vi "playground.vi"() -> ()   [LabVIEW 2014]
panel:
  out "Q Meter":cluster{"Y":dbl[], "Y":dbl[]}[](graph)
  out "Modulator":dynamicdata(graph)
  out "Triangle Waveform":dynamicdata(graph)
  in  "# sweeps":dbl
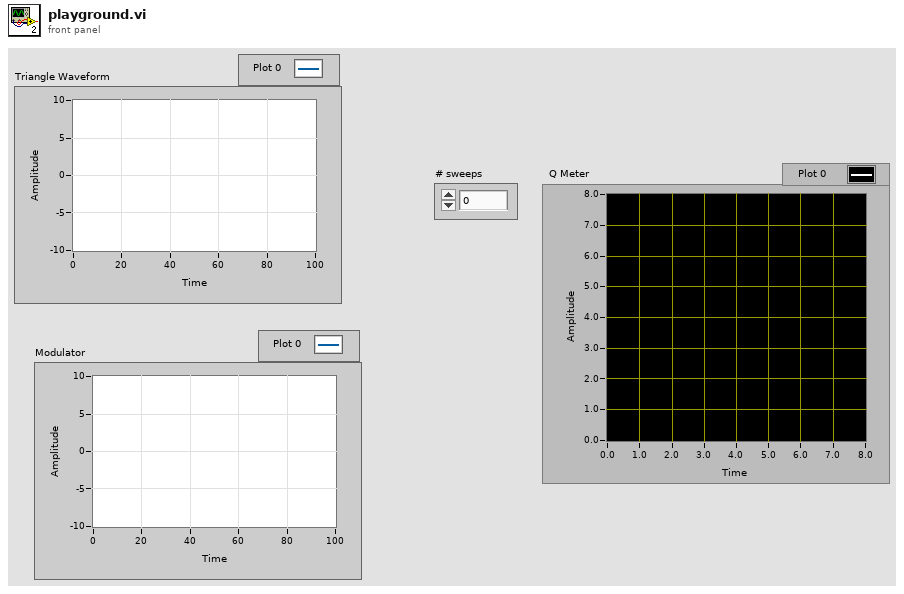
[diagram p1: front panel]
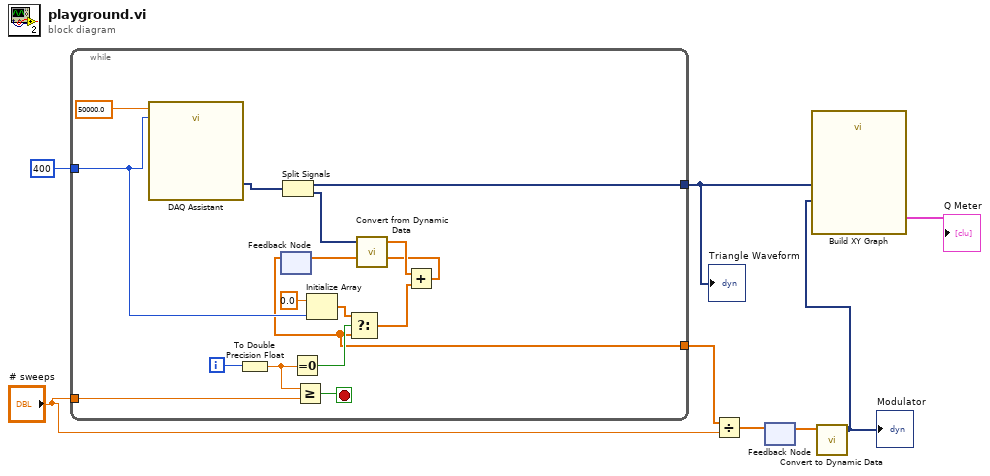
[diagram p0: block diagram]
diagram:
  n1 = while {
    tunnel: 400 -> [w16]
    tunnel: "# sweeps" -> [w12]
    tunnel: [w10] -> w6
    tunnel: [w9] -> w5
    i -> [w15]
    stop <- w13 stop-if-true
    n2 = call "DAQ Assistant"("rate"=50000.0, "number of samples"=w16) -> ("data"=w23:dynamicdata)  [unwired: 15 in, 2 out]
    n3 = To Double Precision Float(number=w15) -> (double precision float=w11:dbl)
    n4 = feedback #1() -> (w9:dbl[])  [unwired: 1 in]
    n5 = Split Signals(w23) -> (w10:dynamicdata, w22:dynamicdata)  [unwired: 2 in]
    n6 = Equal To 0?(x=w11) -> (x = 0?=w14:bool)
    n7 = Greater Or Equal?(x=w11, y=w12) -> (x >= y?=w13:bool)
    n8 = Initialize Array(0.0, w16) -> (w19:dbl[])
    n9 = Select(t=w19, s=w14, f=w9) -> (s? t:f=w17:dbl[])
    n10 = call "Convert from Dynamic Data"("Dynamic Data Type"=w22) -> ("Array"=w21:dbl[])  [unwired: 3 in]
    n11 = Add(x=w21, y=w17) -> (x+y=w20:dbl[])
    n12 = feedback-in #1(w20) -> ()
  }
  "Triangle Waveform" <- w6
  n13 = Divide(x=w5, y="# sweeps") -> (x/y=w3:dbl[])
  n14 = feedback-in #2(w3) -> ()
  n15 = feedback #2() -> (w2:dbl[])  [unwired: 1 in]
  n16 = call "Convert to Dynamic Data"("Array"=w2) -> ("Dynamic Data Type"=w1:dynamicdata)  [unwired: 3 in]
  "Modulator" <- w1
  n17 = call "Build XY Graph"("Y Input"=w1, "X Input"=w6) -> ("XY Graph"=→"Q Meter":cluster{"X":dbl[], "Y":dbl[]}[])  [unwired: 8 in, 1 out]
